vi "tomaData.vi"() -> ()   [LabVIEW 2011]
uses:
  8 - identificacion 3opams/Informe/Programas/Control 1.ctl
panel:
  in  "fs(Hz)":dbl=30.0
  in  "offset":dbl=-0.566
  out "# Muestras":dbl=300.0
  in  "Frecuencia de generador(Hz)":dbl=0.1
  out "Vi":dbl(graph)=4.0787405456815256
  in  "t1(s)":dbl=5.0
  in  "t0(s)":dbl=3.0
  in  "Ring":T1=4 items=["Step"=1, "Gate"=2, "Rampa"=3, "Seno"=4]
  out "salida planta":dynamicdata(graph)=[{"t0"=timestamp(3468875732.713336 s since 1904-01-01), "dt"=1.0, "Y"=[4.0799291610127675]}, {"t0"=timestamp(3468875732.713336 s since 1904-01-01), "dt"=1.0, "Y"=[3.0240292872795367]}]
  out "Vo":dbl=3.0240292872795367
  in  "Amplitud":dbl(slide)=5.0 scale=0.0..5.0
  # "30"
  # "0.1"
  # "300"
  # "t subida"
  # "3000"
  # "5000"
  # "t bajada"
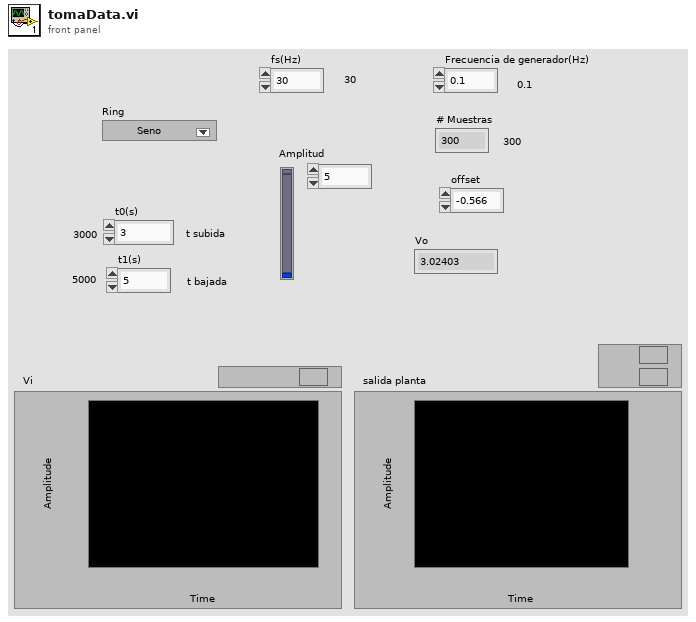
[diagram p1: front panel]
types:
  T1 = typedef "Control 1.ctl" = u16
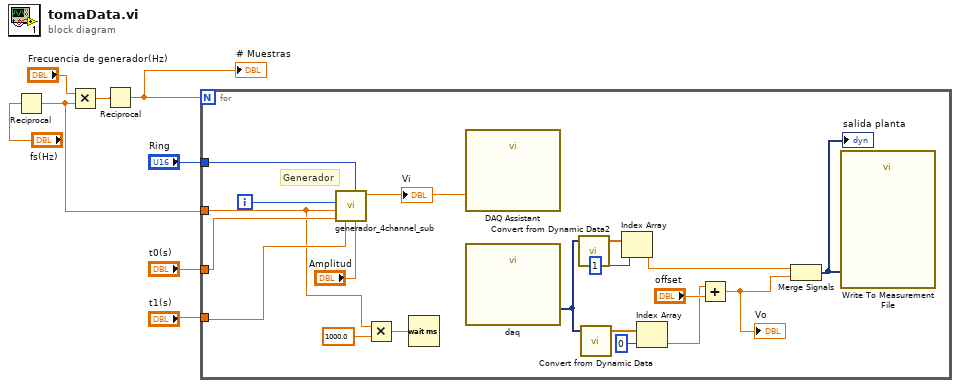
[diagram p0: block diagram]
diagram:
  n1 = Reciprocal(x="fs(Hz)") -> (1/x=w1:dbl)
  n2 = Multiply(x="Frecuencia de generador(Hz)", y=w1) -> (x*y=w5:dbl)
  n3 = Reciprocal(x=w5) -> (1/x=w4:dbl)
  "# Muestras" <- w4
  n4 = for {
    N: w4 -> [_]
    tunnel: "Ring" -> [w27]
    tunnel: w1 -> [w9]
    tunnel: "t0(s)" -> [w26]
    tunnel: "t1(s)" -> [w25]
    i -> [w22]
    # "Generador"
    n5 = call "generador_4channel_sub.vi"("A"="Amplitud", "Ring"=w27, "t1"=w25, "t0"=w26, "T"=w9, "i"=w22) -> ("Waveform Chart"=w23:dbl)  [unwired: 5 in]
    "Vi" <- w23
    n6 = Multiply(x=w9, y=1000.0) -> (x*y=w11:dbl)
    n7 = Wait (ms)(milliseconds to wait=w11) -> ()  [unwired: 1 out]
    n8 = call "DAQ Assistant"("data"=w23) -> ()  [unwired: 17 in, 2 out]
    n9 = call "daq"() -> ("data"=w16:dynamicdata)  [unwired: 17 in, 2 out]
    n10 = call "Convert from Dynamic Data2"("Dynamic Data Type"=w16) -> ("Array"=w19:dbl[])  [unwired: 3 in]
    n11 = call "Convert from Dynamic Data"("Dynamic Data Type"=w16) -> ("Array"=w20:dbl[])  [unwired: 3 in]
    n12 = Index Array(array=w19, index=1) -> (element=w14:dbl)
    n13 = Index Array(array=w20, index=0) -> (element=w15:dbl)
    n14 = Add(x=w15, y="offset") -> (x+y=w13:dbl)
    "Vo" <- w13
    n15 = Merge Signals(w14, w13) -> (w12:dynamicdata)
    "salida planta" <- w12
    n16 = call "Write To Measurement File"("Signals"=w12) -> ()  [unwired: 16 in, 3 out]
  }
